vi "VFH-data_handle-cut_out_part.vi"(7 "Start and stop":i32[](array[numeric]), 11 "data":dbl[](array[numeric])) -> (2 "size(s)":i32, 3 "handled Data":dbl[](array[numeric]))   [LabVIEW 2020, in "VFH-VNA_File_Handler.lvlib"]
uses:
  VFH-VNA_File_Handler.lvlib
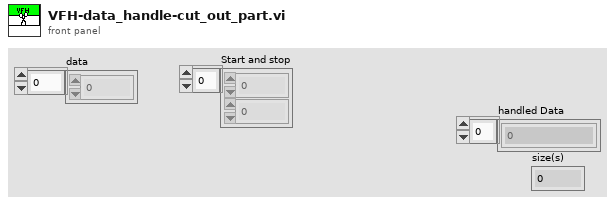
[diagram p1: front panel]
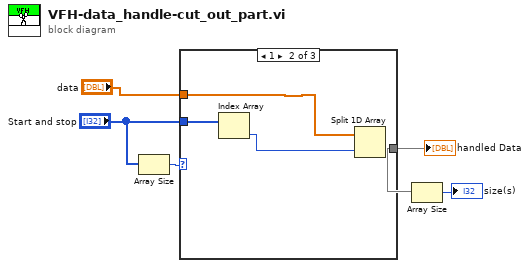
[diagram p0: block diagram]
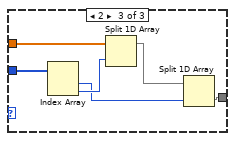
[diagram p3: hidden frame]
diagram:
  n1 = Array Size(array="Start and stop") -> (size(s)=w1:i32)
  n2 = case shown="1" w1 {
    tunnel: "data" -> [w6 w7 w14]
    tunnel: [w6 w9 w12] -> w4
    tunnel: "Start and stop" -> [_ w8 w11]
    frame 0, Default {
    }
    frame 1 {
      n3 = Index Array(array=w8) -> (element=w10:i32)  [unwired: 1 in]
      n4 = Split 1D Array(array=w7, index=w10) -> (second subarray=w9:dbl[])  [unwired: 1 out]
    }
    frame 2 {
      n5 = Index Array(array=w11) -> (element #1=w15:i32, element #2=w16:i32)  [unwired: 2 in]
      n6 = Split 1D Array(array=w14, index=w16) -> (first subarray=w13:dbl[])  [unwired: 1 out]
      n7 = Split 1D Array(array=w13, index=w15) -> (second subarray=w12:dbl[])  [unwired: 1 out]
    }
  }
  "handled Data" <- w4
  n8 = Array Size(array=w4) -> (size(s)=→"size(s)":i32)
